vi "Current_Test_AE.vi"(0 "Current Action":T1, 2 "Action":T2, 7 "Test F(x)":dbl, 11 "Test X":dbl[](array[numeric])) -> (4 "Current Action Out":T1, 8 "Test F(x) Out":dbl, 13 "Reflection F(x)":dbl, 15 "Test X Out":dbl[](array[numeric]))   [LabVIEW 2014]
uses:
  Standard Action.ctl
  Simplex_Engine_Controls.ctl
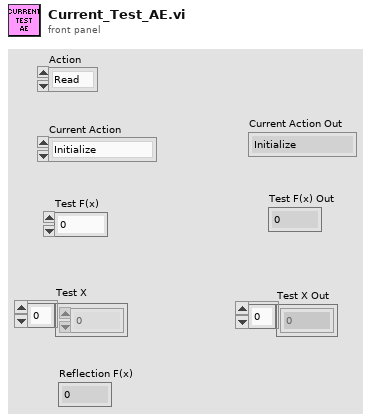
[diagram p1: front panel]
types:
  T1 = typedef "Simplex_Engine_Controls.ctl" = enum16{"Initialize", "Compute Centroid", "Sort", "Evaluate", "Switch", "Get Reflection", "Get Expansion", "Get Contraction", "Get Reduction", "Exit"}
  T2 = typedef "Standard Action.ctl" = enum16{"Read", "Write"}
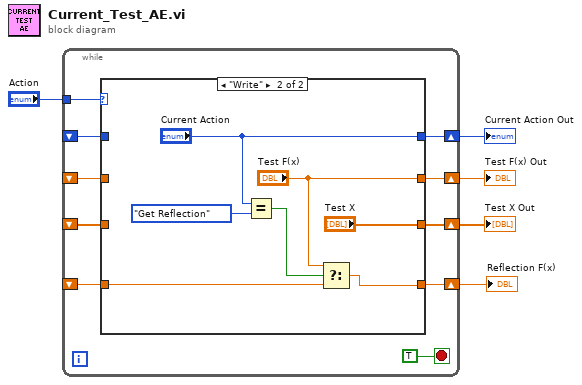
[diagram p0: block diagram]
diagram:
  n1 = while {
    tunnel: "Action" -> [w14]
    shift-right: [w12] -> w4
    shift-left: _ -> [w11]
    shift-right: [w13] -> w3
    shift-left: _ -> [w10]
    shift-right: [w9] -> w2
    shift-left: _ -> [w8]
    shift-right: [w7] -> w1
    shift-left: _ -> [w6]
    stop <- TRUE stop-if-true
    n2 = case shown="\"Write\"" w14 {
      tunnel: [w18 "Test X"] -> w13
      tunnel: [w19 "Current Action"] -> w12
      tunnel: w11 -> [w19 _]
      tunnel: w10 -> [w18 _]
      tunnel: [w17 "Test F(x)"] -> w9
      tunnel: w8 -> [w17 _]
      tunnel: [w16 w21] -> w7
      tunnel: w6 -> [w16 w20]
      frame "Read", Default {
      }
      frame "Write" {
        n3 = Equal?(x="Current Action", y=Simplex_Engine_Controls."Get Reflection") -> (x = y?=w23:bool)
        n4 = Select(t="Test F(x)", s=w23, f=w20) -> (s? t:f=w21:dbl)
      }
    }
  }
  "Current Action Out" <- w4
  "Test X Out" <- w3
  "Test F(x) Out" <- w2
  "Reflection F(x)" <- w1
